vi "Get ObjectType.vi"(8 "error in":errorcluster, 11 "Object Type in":refnum<class "Object Type Base.lvclass">) -> (0 "error out":errorcluster, 1 "Defined?":bool, 2 "ObjectType":T1 items=["UNKNOWN"=255, "NULL"=0, "DOMAIN"=2, "DEFTYPE"=5, "DEFSTRUCT"=6, "VAR"=7, "ARRAY"=8, "RECORD"=9], 3 "Object Type out":refnum<class "Object Type Base.lvclass">)   [LabVIEW 2019, in "Electronic Datasheet.lvlib" / "Object Type Base.lvclass"]
uses:
  Object Type Base.lvclass
  Object Type Base.lvclass/Object Type Base.ctl
  Object Type.ctl
  Electronic Datasheet.lvlib
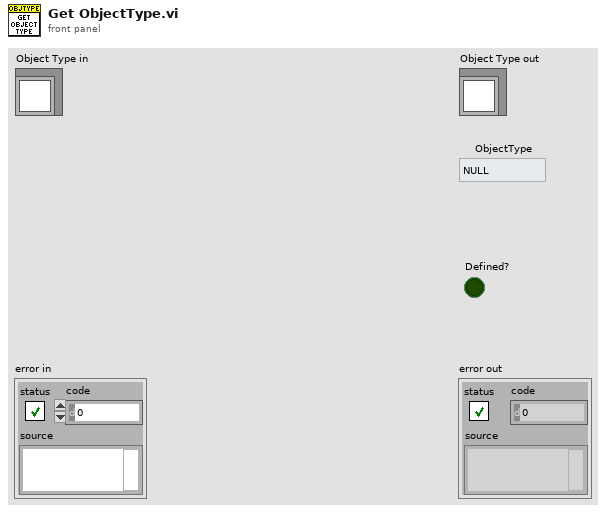
[diagram p1: front panel]
types:
  T1 = typedef "Electronic Datasheet.lvlib/Object Type.ctl" = u8
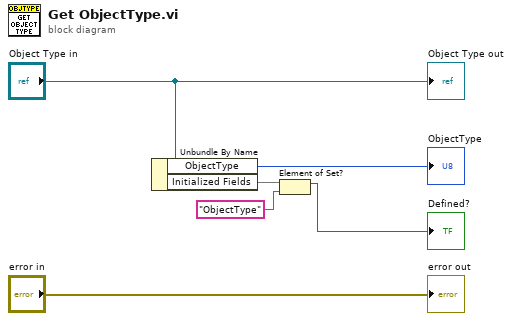
[diagram p0: block diagram]
diagram:
  n1 = Unbundle By Name("Object Type in") -> ("ObjectType"=→"ObjectType":T1, "Initialized Fields"=w3:set{string})
  n2 = Element of Set?(10:"ObjectType" ("element"), 11:w3) -> (3:→"Defined?":bool)
  "error out" <- "error in"
  "Object Type out" <- "Object Type in"
